vi "Get Build Configuration.vi"(6 "Debug Build?":bool, 8 "error in (no error)":errorcluster, 11 "Library Path":path) -> (0 "error out":errorcluster, 2 "Build Config":T1, 3 "Library Path":path)   [LabVIEW 2019, in "PPL INI Parsing.lvlib"]
uses:
  PPL INI Parsing.lvlib
  Build Configuration.ctl
  <vilib>/Utility/config.llb/NI_LVConfig.lvlib
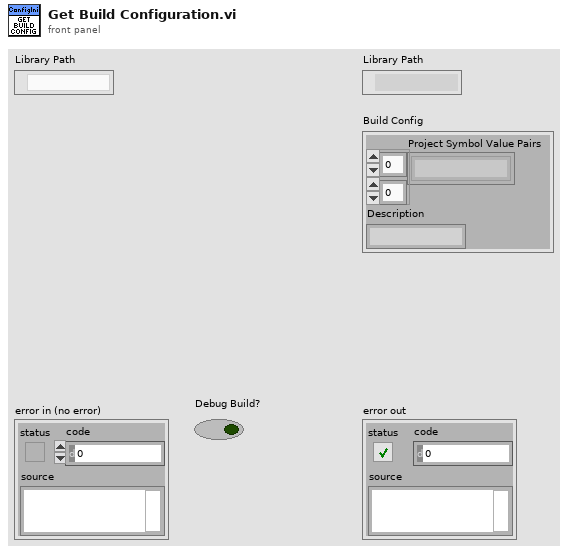
[diagram p1: front panel]
types:
  T1 = typedef "PPL INI Parsing.lvlib/Build Configuration.ctl" = cluster{"SV Pairs":string[][], "Description":string}
  T2 = typedef "NI_LVConfig.lvlib/Config Data RefNum.ctl" = refnum<k1>
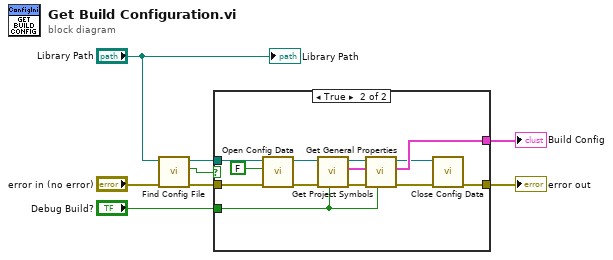
[diagram p0: block diagram]
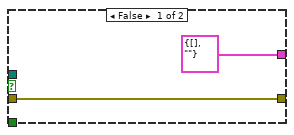
[diagram p2: hidden frame]
diagram:
  n1 = call "Find Config File.vi"("error in (no error)"="error in (no error)", "Library Path"="Library Path") -> ("error out"=w4:errorcluster, "Config File Exists?"=w1:bool, "Ini File Path"=w2:path)  [unwired: 7 in]
  n2 = case shown="True" w1 {
    tunnel: w2 -> [_ w23]
    tunnel: "Debug Build?" -> [_ w11]
    tunnel: [T1 {"SV Pairs"=[], "Description"=""} ("Build Config") w16] -> w6
    tunnel: [w9 w21] -> w5
    tunnel: w4 -> [w9 w20]
    frame False {
    }
    frame True {
      n3 = call <vilib>:"Open Config Data.vi"("error in (no error)"=w20, "create file if necessary (T)"=FALSE, "configuration file path"=w23) -> ("error out"=w18:errorcluster, "refnum"=w19:T2)  [unwired: 6 in, 1 out]
      n4 = call "Get Project Symbols.vi"("Debug Build?"=w11, "error in (no error)"=w18, "Refnum in"=w19) -> ("error out"=w13:errorcluster, "Build Config out"=w17:T1, "Refnum out"=w15:T2)  [unwired: 6 in]
      n5 = call "Get General Properties.vi"("Debug Build?"=w11, "error in (no error)"=w13, "Build Config in"=w17, "Refnum in"=w15) -> ("error out"=w12:errorcluster, "Build Config out"=w16:T1, "Refnum out"=w14:T2)  [unwired: 5 in]
      n6 = call <vilib>:"Close Config Data.vi"("error in (no error)"=w12, "refnum"=w14) -> ("error out"=w21:errorcluster)  [unwired: 8 in, 1 out]
    }
  }
  "Build Config" <- w6
  "error out" <- w5
  "Library Path" <- "Library Path"
